vi "Teardown Framework.vi"(8 "error in (no error)":errorcluster) -> (0 "error out":errorcluster)   [LabVIEW 2023, in "HAF.lvlib"]
doc: "Releases any resources the Framework used. Specifically, it releases events and message queues."
uses:
  HAF.lvlib
  Global Resources.vi
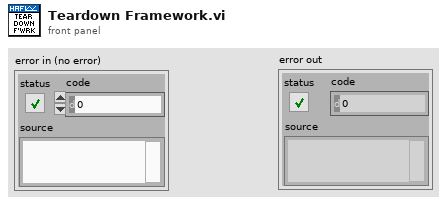
[diagram p1: front panel]
types:
  T1 = typedef "HAF.lvlib/All Message Queues.ctl" = cluster{"Internal":refnum<queue>, "Notifications":refnum<queue>}
  T2 = typedef "HAF.lvlib/All Events.ctl" = cluster{"Stop Event":T3, "Pause":T4, "Resume Event":T5, "Done Event":T6}
  T3 = typedef "HAF.lvlib/Stop Event.ctl" = refnum<user-event>
  T4 = typedef "HAF.lvlib/Pause Event.ctl" = refnum<user-event>
  T5 = typedef "HAF.lvlib/Resume Event.ctl" = refnum<user-event>
  T6 = typedef "HAF.lvlib/Done Event.ctl" = refnum<user-event>
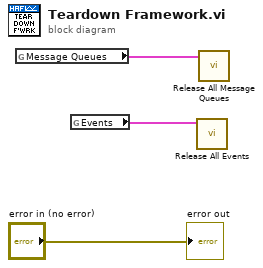
[diagram p0: block diagram]
diagram:
  n1 = global read "Global Resources.vi" "Message Queues"() -> (w3:T1)
  n2 = global read "Global Resources.vi" "Events"() -> (w1:T2)
  n3 = call "Release All Events.vi"("Events"=w1) -> ()  [unwired: 10 in, 1 out]
  n4 = call "Release All Message Queues.vi"("Message Queues"=w3) -> ()  [unwired: 10 in, 1 out]
  "error out" <- "error in (no error)"
